vi "DAQ.vi"(8 "error in":errorcluster, 11 "PID in":refnum<class "INL PID.lvclass">) -> (0 "error out":errorcluster, 2 "Data":dbl[](array[numeric]), 3 "PID out":refnum<class "INL PID.lvclass">)   [LabVIEW 2011, in "INL PID.lvclass"]
uses:
  INL PID.lvclass
  INL PID.lvclass/INL PID.ctl
  <vilib>/DAQmx/read.llb/DAQmx Read (Analog 1D DBL 1Chan NSamp).vi
  <vilib>/DAQmx/miscellaneous.llb/DAQmx Fill In Error Info.vi
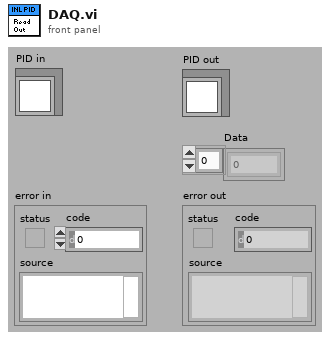
[diagram p1: front panel]
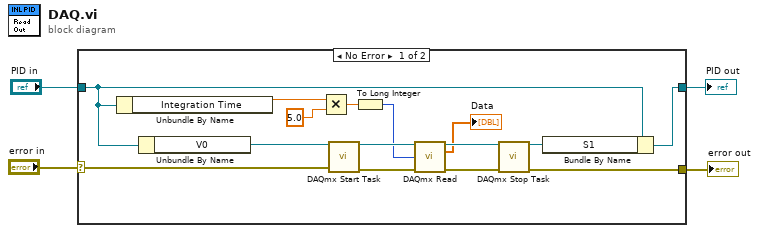
[diagram p0: block diagram]
diagram:
  n1 = case shown="No Error" "error in" {
    selector: "error in" -> [w14 w21]
    tunnel: [w13 w21] -> w3
    tunnel: [w6 w20] -> w1
    tunnel: "PID in" -> [w7 w20]
    frame No Error {
      n2 = Unbundle By Name(w7) -> ("Integration Time"=w5:dbl)
      n3 = Unbundle By Name(w7) -> ("V0"=w15:refnum<k21>)
      n4 = Multiply(x=w5, y=5.0) -> (x*y=w9:dbl)
      n5 = call <vilib>:"DAQmx Start Task.vi"("task/channels in"=w15, "error in"=w14) -> ("task out"=w16:refnum<k21>, "error out"=w17:errorcluster)  [unwired: 12 in]
      n6 = To Long Integer(number=w9) -> (32bit integer=w8:i32)
      n7 = call-poly <vilib>:"DAQmx Read.vi"("task/channels in"=w16, "number of samples per channel"=w8, "error in"=w17) -> ("task out"=w18:refnum<k21>, "data"=→"Data":dbl[], "error out"=w19:errorcluster)  [unwired: 10 in]
      n8 = call <vilib>:"DAQmx Stop Task.vi"("task/channels in"=w18, "error in"=w19) -> ("task out"=w11:refnum<k21>, "error out"=w13:errorcluster)  [unwired: 12 in]
      n9 = Bundle By Name(cluster=w7, "S1"=w11) -> (w6:refnum<class "INL PID.lvclass">)
    }
    frame Error {
    }
  }
  "error out" <- w3
  "PID out" <- w1
